vi "monochromatorCommandSetWavelength.vi"(8 "error in":errorcluster, 10 "wavelength":dbl, 11 "monochromator":refnum<k24>) -> (0 "error out":errorcluster, 2 "wavelength set":bool, 3 "monochromator":refnum<k24>)   [LabVIEW 2009]
doc: "Send Monochromator to requested wavelength"
uses:
  C:/Users/anderson.chen/Desktop/Software Development/Cornerstone Series API (LV9)/Cornerstone DLL/Cornerstone.dll
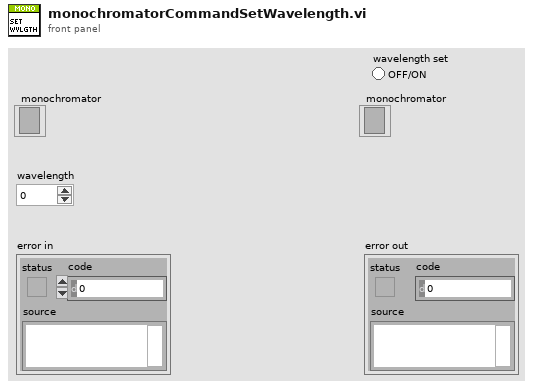
[diagram p1: front panel]
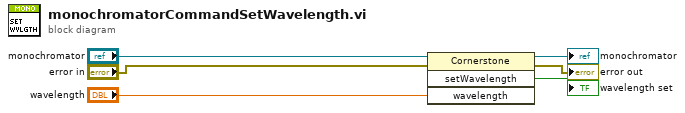
[diagram p0: block diagram]
diagram:
  n1 = invoke class="Cornerstone" method="setWavelength"(reference="monochromator", error in="error in", "wavelength"="wavelength") -> (reference out=→"monochromator":refnum<k24>, error out=→"error out":errorcluster, "setWavelength"=→"wavelength set":bool)  [unwired: 1 in, 1 out]
